vi "Wait for First Request.vi"(8 "error in (no error)":errorcluster, 10 "Elevator Location":T1, 11 "Elevator Controller Actor in":refnum<class "Elevator Controller Actor.lvclass">) -> (0 "error out":errorcluster, 3 "Elevator Controller Actor out":refnum<class "Elevator Controller Actor.lvclass">)   [LabVIEW 2019, in "Elevator Controller Actor.lvlib" / "Elevator Controller Actor.lvclass"]
uses:
  Elevator Controller Actor.lvclass
  Elevator Controller Actor Messages/Set State Msg/Set State Msg.lvclass
  State -Enum.ctl
  Sim Display Console Actor/Elevator Controller/Floor -Enum.ctl
  Sim Display Console Actor/Elevator Controller/Sim Display Console Actor.lvclass
  <vilib>/ActorFramework/Actor/Actor.lvclass
  C:/Program Files (x86)/National Instruments/LabVIEW 2019/vi.lib/ActorFramework/Actor/Actor.lvclass
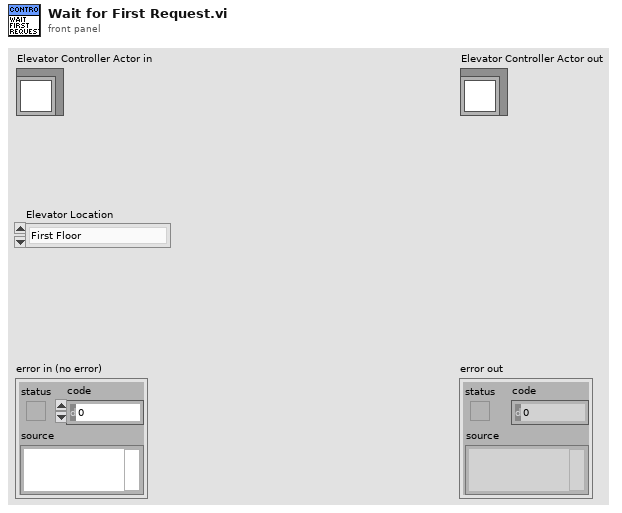
[diagram p1: front panel]
types:
  T1 = typedef "Simulated Display Console Actor.lvlib/Sim Display Console Actor.lvclass/Floor -Enum.ctl" = enum16{"First Floor", "Send Floor", "Third Floor", "Fourth Floor"}
  T2 = typedef "Elevator Controller Actor.lvlib/Elevator Controller Actor.lvclass/State -Enum.ctl" = enum16{"Initial", "Wait for First Request", "Start and Move", "Anaysis", "Continue Travel", "Stop at Floor", "Open and Close Door Sequence", "No Request Remaining", "Emergency Call", "Terminate Process"}
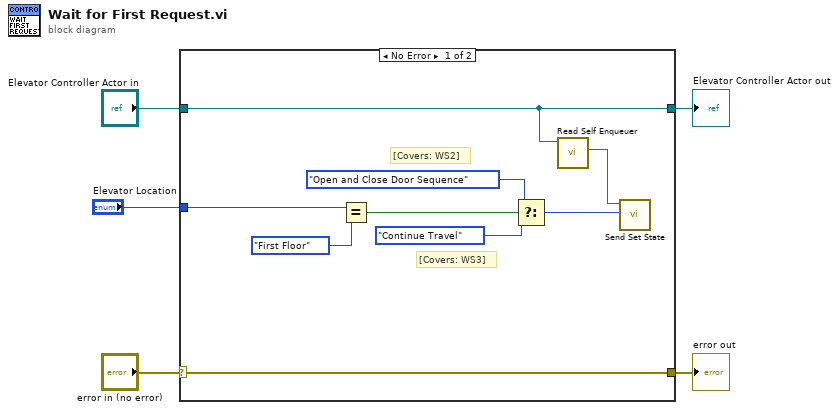
[diagram p0: block diagram]
diagram:
  n1 = case shown="No Error" "error in (no error)" {
    selector: "error in (no error)" -> [w7 w16]
    tunnel: [w7 w16] -> w4
    tunnel: [w9 w15] -> w2
    tunnel: "Elevator Controller Actor in" -> [w9 w15]
    tunnel: "Elevator Location" -> [w6 _]
    frame No Error {
      # "[Covers: WS3]"
      # "[Covers: WS2]"
      n2 = Equal?(x=w6, y=Floor_-Enum."First Floor") -> (x = y?=w11:bool)
      n3 = Select(t=State_-Enum."Open and Close Door Sequence" ("States"), s=w11, f=State_-Enum."Continue Travel" ("States")) -> (s? t:f=w12:T2)
      n4 = call <vilib>:"Read Self Enqueuer.vi"("Actor"=w9) -> ("Self Enqueuer"=w8:refnum<class "Message Enqueuer.lvclass">)  [unwired: 10 in]
      n5 = call "Send Set State.vi"("States"=w12, "Message Enqueuer"=w8) -> ()  [unwired: 8 in, 2 out]
    }
    frame Error {
    }
  }
  "error out" <- w4
  "Elevator Controller Actor out" <- w2
